vi "Configure Current Limit.vi"(6 "Settle (1mS)":u32=1, 8 "error in (no error)":errorcluster, 10 "Current Limit (0A)":dbl format="%.4f", 11 "VISA resource name":refnum<visa-resource-name>) -> (0 "error out":errorcluster, 3 "VISA resource name out":refnum<visa-resource-name>)   [LabVIEW 2020, in "TDK-Lambda Z.lvlib"]
doc: "Configures the current limit. The power supply output will go to this limit if the load causes Constant-Current operation.\n\nNote: This VI will wait for \"Settle\" milliseconds after setting the limit to allow the output to reach the new setting. If unwired, there will be no delay"
uses:
  TDK-Lambda Z.lvlib
panel:
  out "Response":string
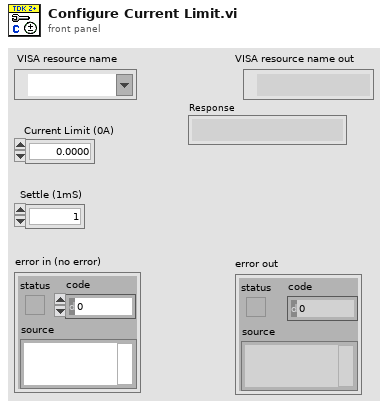
[diagram p1: front panel]
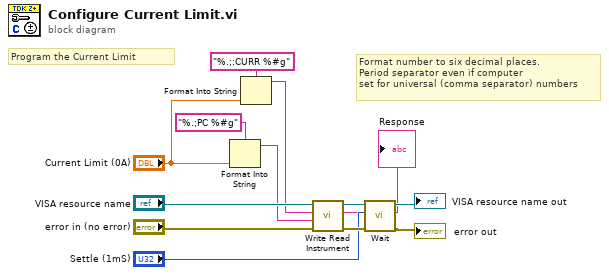
[diagram p0: block diagram]
diagram:
  # "Format number to six decimal places.\nPeriod separator even if computer \nset for universal (comma separator) numbers"
  # "Program the Current Limit"
  n1 = Format Into String(format string="%.;PC %#g", "Current Limit (0A)") -> (resulting string=w8:string)  [unwired: 2 in, 1 out]
  n2 = Format Into String(format string="%.;:CURR %#g", "Current Limit (0A)") -> (resulting string=w11:string)  [unwired: 2 in, 1 out]
  n3 = call "Write Read Instrument.vi"("error in (no error)"="error in (no error)", "GEN  Write Command/Query"=w8, "SCPI  Write Command/Query"=w11, "VISA resource name"="VISA resource name") -> ("error out"=w5:errorcluster, "Response"=→"Response":string, "VISA resource name out"=w6:refnum<visa-resource-name>)  [unwired: 5 in]
  n4 = call "Wait.vi"("error in (no error)"=w5, "Wait (1mS)"="Settle (1mS)", "VISA resource name"=w6) -> ("error out"=→"error out":errorcluster, "VISA resource name out"=→"VISA resource name out":refnum<visa-resource-name>)  [unwired: 7 in]
